vi "Wait on SRQ.vi"(8 "error in (no error)":errorcluster {"code" format="%.0x"}, 11 "VISA session":refnum<visa-resource-name>) -> (0 "error out":errorcluster {"code" format="%.0x"}, 3 "dup VISA session":refnum<visa-resource-name>)   [LabVIEW 2011]
doc: "Waits on a service request, discards any events already in the queue, then enables VISA event handling for a service request.\n\nThis VI is part of an SRQ operation sequence, the order of which is as follows:\n\n1) Set up instrument event enable registers\n2) Call Initialize SRQ.vi\n3) Perform an operation that causes the instrument to generate a service request\n4) Call Wait on SRQ.vi\n\nUse the following VIs to help you set up the instrument event-enable registers: \n\nSet-Query SRER.vi\nSet-Query SESER.vi\nOther instrument-specific event-enable registers (e.g., Agilent 34401A Questionable Data Event Register)\n\nNote: Use this VI as an optional replacement to calling Wait for RQS.vi followed by a VISA Disable Event."
uses:
  <vilib>/Instr/_visa.llb/Select Event Type.ctl
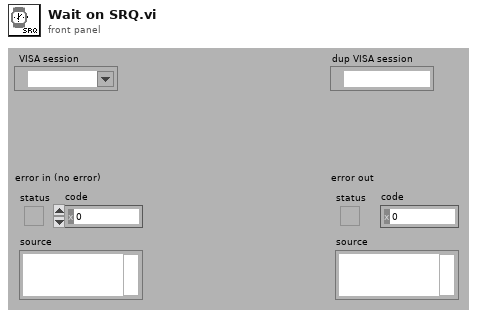
[diagram p1: front panel]
types:
  T1 = typedef "Select Event Type.ctl" = u32
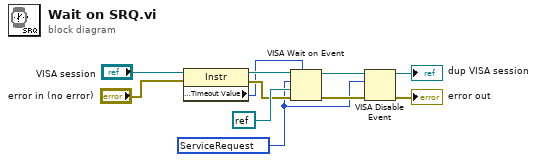
[diagram p0: block diagram]
diagram:
  w5 = T1 1073684491 items=["ServiceRequest"=1073684491, "Trigger"=3221168138, "Clear"=1073684493, "VXI-Signal"=1073684512, "VXI/VME-Interrupt"=3221168161, "VXI/VME-Sysfail"=1073684509, "VXI/VME-Sysreset"=1073684510, "GPIB-CIC"=1073684498, "GPIB-Talk"=1073684499, "GPIB-Listen"=1073684500, "PXI-Interrupt"=1073684514, "AllEnabled"=1073709055] ("Event Type")
  n1 = property class="Instr"(reference="VISA session", error in="error in (no error)") -> (reference out=w10:refnum<visa-resource-name>, error out=w9:errorcluster, "General Settings:Timeout Value"=w6:u32)
  n2 = VISA Wait on Event(7:w6, 8:w9, 9:refnum<visa-resource-name> refnum ("event resource class"), 10:w5, 11:w10) -> (0:w7:errorcluster, 3:w8:refnum<visa-resource-name>)  [unwired: 2 out]
  n3 = VISA Disable Event(8:w7, 10:w5, 11:w8) -> (0:→"error out":errorcluster, 3:→"dup VISA session":refnum<visa-resource-name>)  [unwired: 1 in]
